vi "Update Runtime Error Indicator.vi"(8 "error in (no error)":errorcluster, 10 "Error Count":u32, 11 "Cfg Grandmaster in":refnum<class "Cfg Grandmaster.lvclass">) -> (0 "error out":errorcluster, 3 "Cfg Grandmaster out":refnum<class "Cfg Grandmaster.lvclass">)   [LabVIEW 2012, in "Configuration Grandmaster.lvlib" / "Cfg Grandmaster.lvclass"]
uses:
  Cfg Grandmaster.lvclass
  Cfg Grandmaster.lvclass/Cfg Grandmaster.ctl
  Class FP Ctrls/FP Controls.lvclass
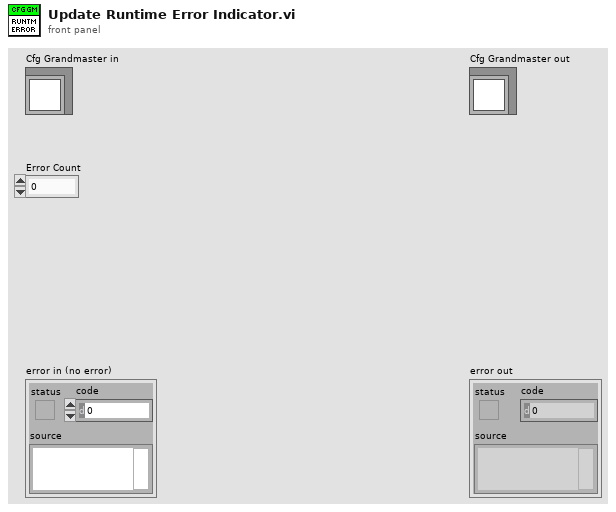
[diagram p1: front panel]
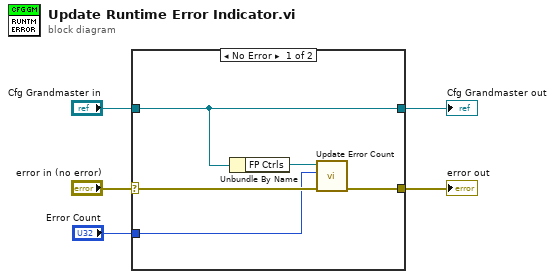
[diagram p0: block diagram]
diagram:
  n1 = case shown="No Error" "error in (no error)" {
    selector: "error in (no error)" -> [w8 w12]
    tunnel: [w7 w12] -> w4
    tunnel: [w10 w11] -> w2
    tunnel: "Cfg Grandmaster in" -> [w10 w11]
    tunnel: "Error Count" -> [w6 _]
    frame No Error {
      n2 = Unbundle By Name(w10) -> ("FP Ctrls"=w9:refnum<class "FP Controls.lvclass">)
      n3 = call "Update Error Count.vi"("error in (no error)"=w8, "Error Count"=w6, "FP Controls in"=w9) -> ("error out"=w7:errorcluster)  [unwired: 7 in, 1 out]
    }
    frame Error {
    }
  }
  "error out" <- w4
  "Cfg Grandmaster out" <- w2
